vi "Write to Log Videos.vi"(6 "AVI Refnum":T1, 7 "New Image":T2, 8 "error in (no error)":errorcluster, 9 "Session Out":T3="cam0", 10 "Array of Waveforms":waveform(dbl)[](array[waveform]), 11 "Log File in":refnum<k34>) -> (0 "error out":errorcluster, 3 "Log File out":refnum<k34>)   [LabVIEW 2017]
uses:
  <vilib>/userdefined/High Color/IMAQdx.ctl
  <vilib>/vision/Image Controls.llb/IMAQ Image.ctl
  <vilib>/vision/Avi.llb/IMAQ AVI2 Refnum.ctl
  <vilib>/vision/Avi.llb/IMAQ AVI2 Codec Path.ctl
  <vilib>/vision/driver/NI_Vision_Acquisition_Software.lvlib
panel:
  out "Webcam":T2(plugin-control)
  in  "stop":bool
  out "Codec Names":string[](array[string])
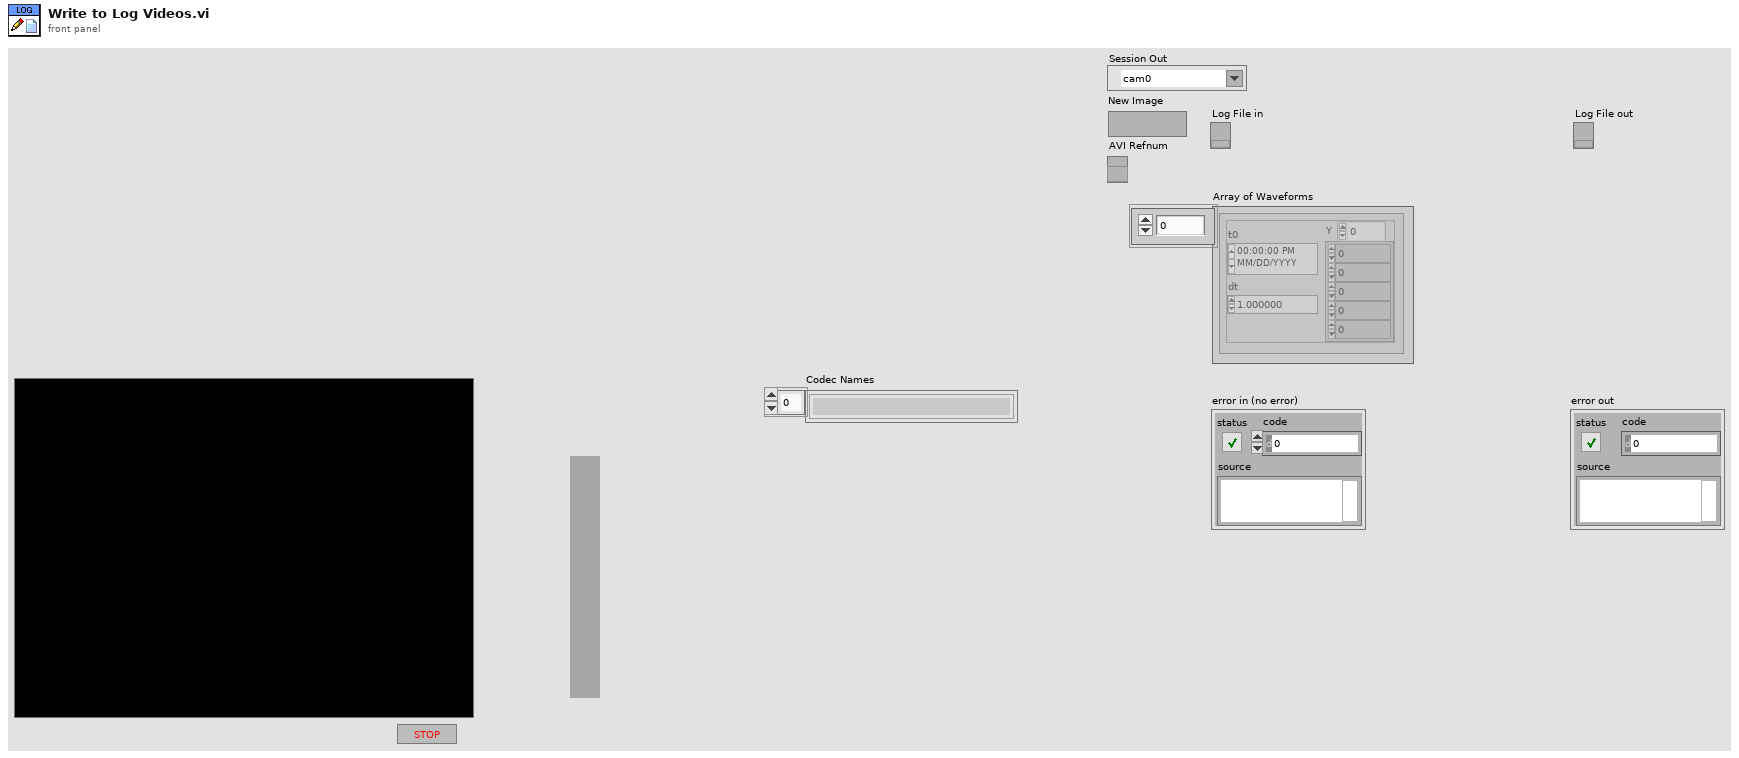
[diagram p1: front panel]
types:
  T1 = typedef "IMAQ AVI2 Refnum.ctl" = refnum<k20>
  T2 = typedef "IMAQ Image.ctl" = refnum<image>
  T3 = typedef "IMAQdx.ctl" = refnum<k21>
  T4 = typedef "IMAQ AVI2 Codec Path.ctl" = u32
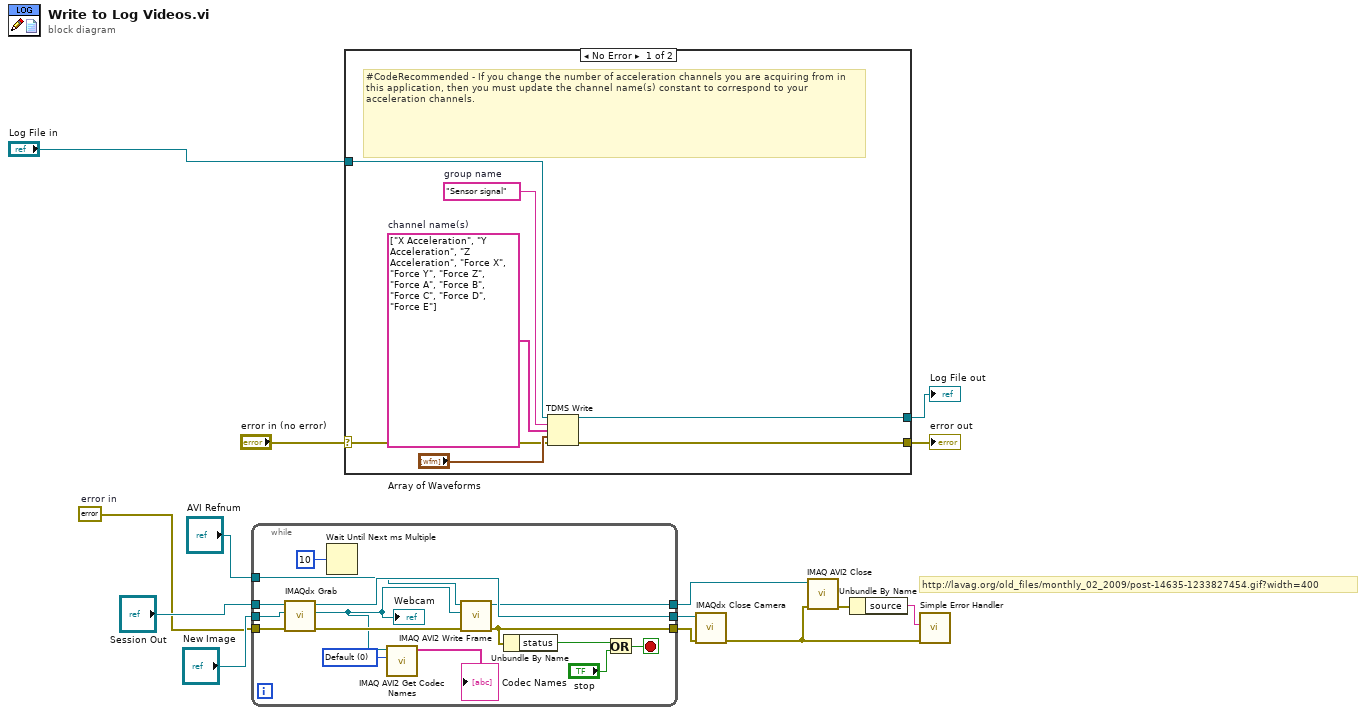
[diagram p0: block diagram]
diagram:
  w1 = errorcluster {"status"=FALSE, "code"=0, "source"=""}  # error in
  # "http://lavag.org/old_files/monthly_02_2009/post-14635-1233827454.gif?width=400"
  n1 = while {
    tunnel: w1 -> [w29]
    tunnel: "Session Out" -> [w28]
    tunnel: "New Image" -> [w27]
    tunnel: [w21] -> w10
    tunnel: [w26] -> w9
    tunnel: "AVI Refnum" -> [w24]
    tunnel: [w23] -> w5
    stop <- w18 stop-if-true
    w16 = T4 0 items=["Default", "System", "Built in Vision"] ("Codec Source")
    n2 = call <vilib>:"IMAQdx Grab.vi"("error in"=w29, "Image In"=w27, "Session In"=w28) -> ("error out"=w22:errorcluster, "Image Out"=w17:T2, "Session Out"=w26:T3)  [unwired: 5 in, 1 out]
    "Webcam" <- w17
    n3 = Wait Until Next ms Multiple(millisecond multiple=u32 10 ("milliseconds to wait")) -> ()  [unwired: 1 out]
    n4 = call "IMAQ AVI2 Get Codec Names"("Codec Source"=w16, "Image"=w17) -> ("Codec Names"=→"Codec Names":string[])  [unwired: 8 in, 1 out]
    n5 = call "IMAQ AVI2 Write Frame"("error in (no error)"=w22, "Image"=w17, "AVI Refnum"=w24) -> ("error out"=w21:errorcluster, "AVI Refnum (duplicate)"=w23:T1)  [unwired: 6 in, 1 out]
    n6 = Unbundle By Name(w21) -> ("status"=w20:bool)
    n7 = Or(x=w20, y="stop") -> (x .or. y?=w18:bool)
  }
  n8 = case shown="No Error" "error in (no error)" {
    selector: "error in (no error)" -> [w31 w37]
    tunnel: "Log File in" -> [w33 w38]
    tunnel: [w32 w38] -> w13
    tunnel: [w30 w37] -> w11
    frame No Error {
      w34 = string[] ["X Acceleration", "Y Acceleration", "Z Acceleration", "Force X", "Force Y", "Force Z", "Force A", "Force B", "Force C", "Force D", "Force E"]  # channel name(s)
      w36 = "Sensor signal"  # group name
      # "#CodeRecommended - If you change the number of acceleration channels you are acquiring from in this application, then you must update the channel name(s) constant to correspond to your acceleration channels."
      n9 = TDMS Write(0:w33, 5:w36, 7:w34, 9:"Array of Waveforms", 11:w31) -> (4:w32:refnum<k34>, 15:w30:errorcluster)  [unwired: 1 in, 2 out]
    }
    frame Error {
    }
  }
  "Log File out" <- w13
  "error out" <- w11
  n10 = call <vilib>:"IMAQdx Close Camera.vi"("error in"=w10, "Session In"=w9) -> ("error out"=w7:errorcluster)  [unwired: 9 in]
  n11 = call "IMAQ AVI2 Close"("error in (no error)"=w7, "AVI Refnum"=w5) -> ("error out"=w6:errorcluster)  [unwired: 9 in]
  n12 = Unbundle By Name(w6) -> ("source"=w8:string)
  n13 = call <vilib>:"Simple Error Handler.vi"("error source (\" \")"=w8, "error in (no error)"=w7) -> ()  [unwired: 3 in, 5 out]
